vi "Receive Read Bit Data.vi"(8 "error in (no error)":errorcluster, 11 "Port Selection Info":T1={"Port Name"="", "Amplifier Num"=1, "Baud Rate"=38400, "Char Formation"=enum."0"} {"Baud Rate" items=["38400"=38400, "19200"=19200, "9600"=9600, "115200"=0]; "Amplifier Num" max=31}) -> (0 "error out":errorcluster, 1 "bits array":bool[](array[boolean]), 2 "byte num":u8, 3 "Port Selection Info Out":T1={"Port Name"="", "Amplifier Num"=1, "Baud Rate"=38400, "Char Formation"=enum."0"} {"Baud Rate" items=["38400"=38400, "19200"=19200, "9600"=9600, "115200"=0]; "Amplifier Num" max=31}, 4 "CRC Match":bool, 5 "FC":u8, 7 "Bank":u8)   [LabVIEW 2014, in "ALPHA5 RS485.lvlib"]
uses:
  ALPHA5 RS485.lvlib
  typedefs/Port Selection Info.ctl
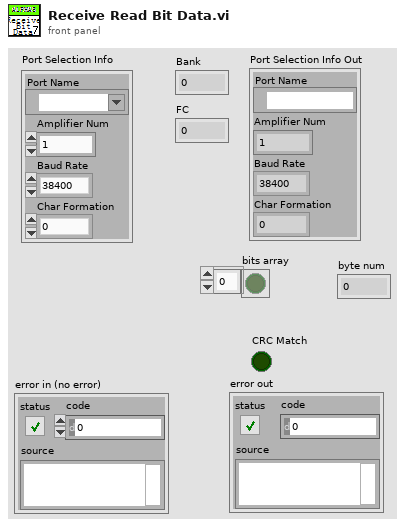
[diagram p1: front panel]
types:
  T1 = typedef "ALPHA5 RS485.lvlib/Port Selection Info.ctl" = cluster{"Port Name":refnum<visa-resource-name>, "Amplifier Num":u8, "Baud Rate":u32, "Char Formation":enum16{"0", "1", "2", "3", "4", "5"}}
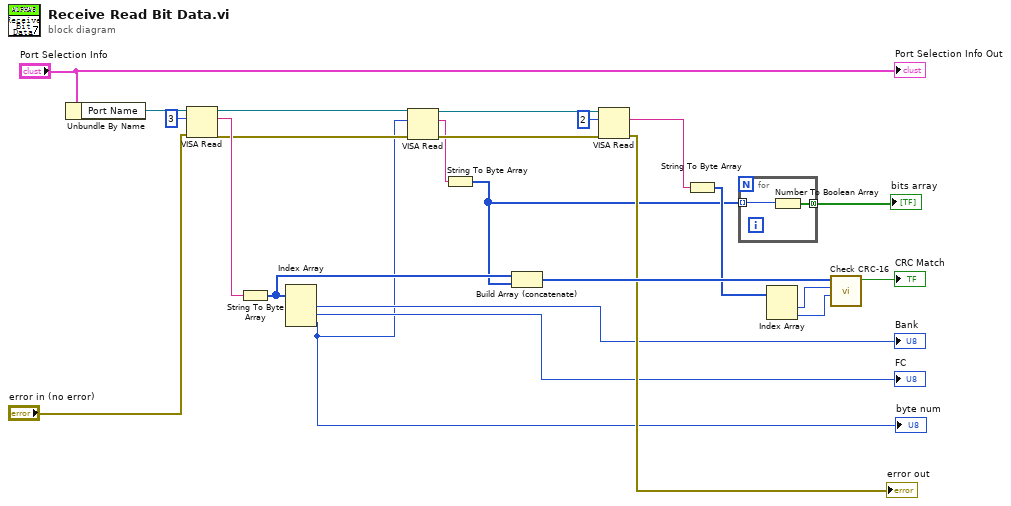
[diagram p0: block diagram]
diagram:
  n1 = Unbundle By Name("Port Selection Info") -> ("Port Name"=w23:refnum<visa-resource-name>)
  n2 = VISA Read(VISA resource name=w23, byte count=u32 3, error in (no error)="error in (no error)") -> (VISA resource name out=w19:refnum<visa-resource-name>, read buffer=w20:string, error out=w18:errorcluster)  [unwired: 1 out]
  n3 = String To Byte Array(string=w20) -> (unsigned byte array=w14:u8[])
  n4 = Index Array(array=w14) -> (element #1=→"Bank":u8, element #2=→"FC":u8, element #3=w3:u8)  [unwired: 3 in]
  "byte num" <- w3
  n5 = VISA Read(VISA resource name=w19, byte count=w3, error in (no error)=w18) -> (VISA resource name out=w17:refnum<visa-resource-name>, read buffer=w13:string, error out=w16:errorcluster)  [unwired: 1 out]
  n6 = String To Byte Array(string=w13) -> (unsigned byte array=w2:u8[])
  n7 = Build Array (concatenate)(w14, w2) -> (w12:u8[])
  n8 = VISA Read(VISA resource name=w17, byte count=u32 2, error in (no error)=w16) -> (read buffer=w11:string, error out=→"error out":errorcluster)  [unwired: 2 out]
  n9 = String To Byte Array(string=w11) -> (unsigned byte array=w10:u8[])
  n10 = for {
    tunnel: w2 -> [w26] mode=indexing
    tunnel: [w25] -> w1 mode=concatenating
    n11 = Number To Boolean Array(number=w26) -> (Boolean array=w25:bool[])
  }
  "bits array" <- w1
  n12 = Index Array(array=w10) -> (element #1=w8:u8, element #2=w9:u8)  [unwired: 2 in]
  n13 = call "Check CRC-16.vi"("CRC-16-H"=w9, "CRC-16-L"=w8, "Data In"=w12) -> ("Check Result"=→"CRC Match":bool)  [unwired: 7 in, 1 out]
  "Port Selection Info Out" <- "Port Selection Info"
